vi "ProducerConsumerData (Multiple Queue Array).vi"() -> ()   [LabVIEW 2019]
doc: "Use this template to build a producer/consumer design pattern. Use this template when you need to execute a process, such as data analysis, when a data source, such as a triggered acquisition, produces data at an uneven rate and you need to execute the process when the data becomes available."
panel:
  out "data (can be any type) 2":string
  out "data (can be any type)":string
  in  "stop":bool
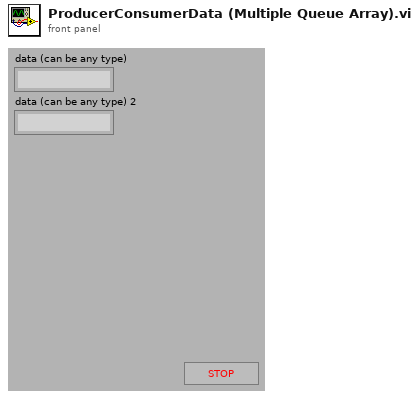
[diagram p1: front panel]
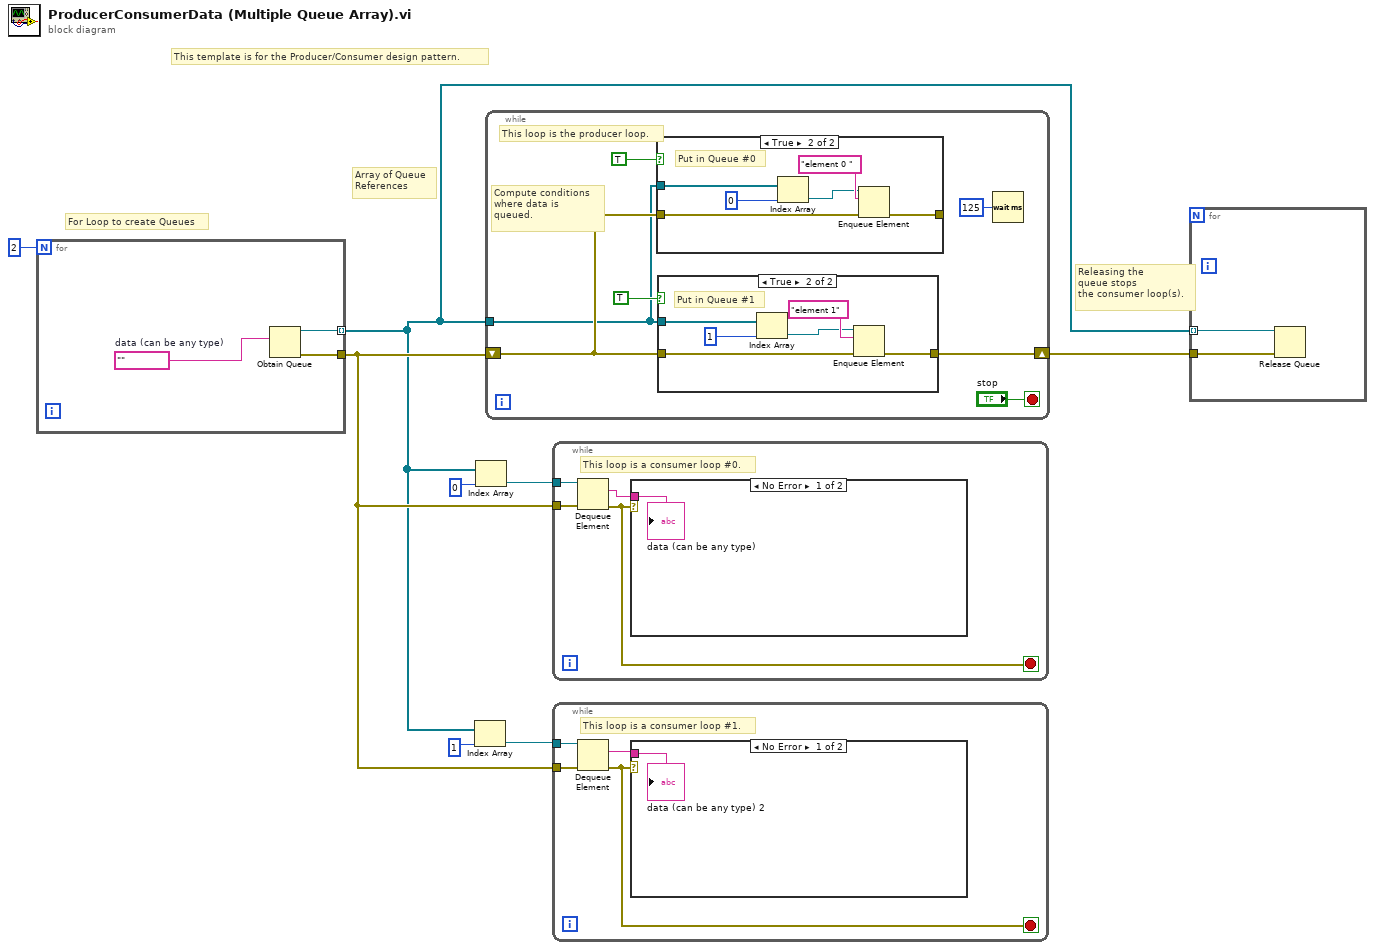
[diagram p0: block diagram]
diagram:
  # "Array of Queue\nReferences"
  # "For Loop to create Queues"
  # "Releasing the\nqueue stops\nthe consumer loop(s)."
  # "This template is for the Producer/Consumer design pattern."
  n1 = for {
    N: 2 -> [_]
    tunnel: [w11] -> w3
    tunnel: [w9] -> w1 mode=indexing
    w10 = ""  # data (can be any type)
    n2 = Obtain Queue(element data type=w10) -> (queue out=w9:refnum<queue>, error out=w11:errorcluster)  [unwired: 4 in, 1 out]
  }
  n3 = Index Array(array=w1, index=1) -> (element=w2:refnum<queue>)
  n4 = Index Array(array=w1, index=0) -> (element=w5:refnum<queue>)
  n5 = while {
    shift-right: [w13] -> w7
    shift-left: w3 -> [w14]
    tunnel: w1 -> [w12]
    stop <- "stop" stop-if-true
    # "Compute conditions\nwhere data is\nqueued."
    # "This loop is the producer loop."
    n6 = case shown="True" TRUE {
      tunnel: [w19 w25] -> _
      tunnel: w14 -> [w19 w21]
      tunnel: w12 -> [_ w22]
      frame False {
      }
      frame True {
        # "Put in Queue #0"
        n7 = Index Array(array=w22, index=0) -> (element=w20:refnum<queue>)
        n8 = Enqueue Element(queue=w20, element="element 0 ", error in (no error)=w21) -> (error out=w25:errorcluster)  [unwired: 1 in, 2 out]
      }
    }
    n9 = case shown="True" TRUE ("Case Constant\n(See Context Help)") {
      tunnel: w14 -> [w26 w28]
      tunnel: [w26 w32] -> w13
      tunnel: w12 -> [_ w29]
      frame False {
      }
      frame True {
        # "Put in Queue #1"
        n10 = Index Array(array=w29, index=1) -> (element=w30:refnum<queue>)
        n11 = Enqueue Element(queue=w30, element="element 1", error in (no error)=w28) -> (error out=w32:errorcluster)  [unwired: 1 in, 2 out]
      }
    }
    n12 = Wait (ms)(milliseconds to wait=u32 125) -> ()  [unwired: 1 out]
  }
  n13 = while {
    tunnel: w5 -> [w36]
    tunnel: w3 -> [w34]
    stop <- w35 stop-if-true
    # "This loop is a consumer loop #0."
    n14 = Dequeue Element(queue=w36, error in (no error)=w34) -> (element=w33:string, error out=w35:errorcluster)  [unwired: 1 in, 2 out]
    n15 = case shown="No Error" w35 {
      tunnel: w33 -> [w37 _]
      frame No Error {
        "data (can be any type)" <- w37
      }
      frame Error {
      }
    }
  }
  n16 = while {
    tunnel: w2 -> [w40]
    tunnel: w3 -> [w39]
    stop <- w41 stop-if-true
    # "This loop is a consumer loop #1."
    n17 = Dequeue Element(queue=w40, error in (no error)=w39) -> (element=w38:string, error out=w41:errorcluster)  [unwired: 1 in, 2 out]
    n18 = case shown="No Error" w41 {
      tunnel: w38 -> [w42 _]
      frame No Error {
        "data (can be any type) 2" <- w42
      }
      frame Error {
      }
    }
  }
  n19 = for {
    tunnel: w7 -> [w44]
    tunnel: w1 -> [w43] mode=indexing
    n20 = Release Queue(queue=w43, error in (no error)=w44) -> ()  [unwired: 1 in, 3 out]
  }
